vi "Insert Element at Index.vi"(6 "index":i32, 8 "error in (no error)":errorcluster, 9 "element":variant, 10 "Name":string, 11 "Cluster in":variant) -> (0 "error out":errorcluster, 3 "Cluster out":variant)   [LabVIEW 2017, in "Variant Data Manipulation.lvlib"]
uses:
  Variant Data Manipulation.lvlib
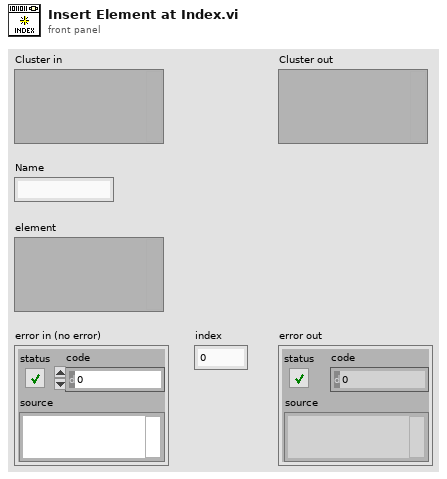
[diagram p1: front panel]
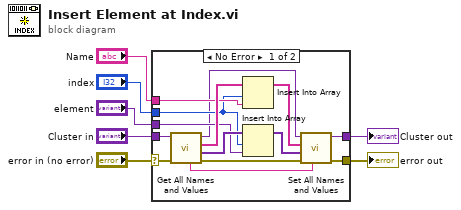
[diagram p0: block diagram]
diagram:
  n1 = case shown="No Error" "error in (no error)" {
    selector: "error in (no error)" -> [w21 w22]
    tunnel: [w19 w22] -> w6
    tunnel: [w18 w23] -> w5
    tunnel: "Cluster in" -> [w17 w23]
    tunnel: "Name" -> [w15 _]
    tunnel: "index" -> [w12 _]
    tunnel: "element" -> [w11 _]
    frame No Error {
      n2 = call "Get All Names and Values.vi"("error in"=w21, "Cluster in"=w17) -> ("error out"=w20:errorcluster, "Values"=w13:variant[], "Element Names"=w16:string[], "Cluster out"=w8:variant, "Cluster Name"=w9:string)  [unwired: 5 in]
      n3 = Insert Into Array(array=w16, index=w12, new element=w15) -> (w14:string[])
      n4 = Insert Into Array(array=w13, index=w12, new element=w11) -> (w10:variant[])
      n5 = call "Set All Names and Values.vi"("Cluster Name"=w9, "error in"=w20, "values"=w10, "Element Names"=w14, "Cluster in"=w8) -> ("error out"=w19:errorcluster, "Cluster out"=w18:variant)  [unwired: 5 in]
    }
    frame Error {
    }
  }
  "Cluster out" <- w5
  "error out" <- w6
